vi "Resize Bounds.vi"(10 "Resize Amount":i16, 11 "Bounds In":T1) -> (3 "Bounds Out":T1)   [LabVIEW 2019, in "2D.lvlib"]
doc: "Resizes the bounding rectangle by the given amount. All edges of the rectangle will be changed by the Resize Amount. For example a resizing a bounding rectangle of [0,0,100,100] by 8 will result in a [-8,-8,108,108] bounding rectangle."
uses:
  <vilib>/Utility/miscctls.llb/LVRectTypeDef.ctl
  2D.lvlib
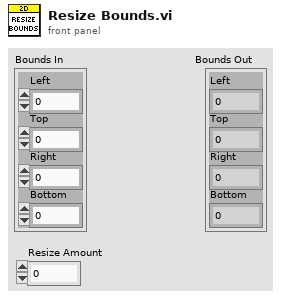
[diagram p1: front panel]
types:
  T1 = typedef "LVRectTypeDef.ctl" = cluster{"Left":i16, "Top":i16, "Right":i16, "Bottom":i16}
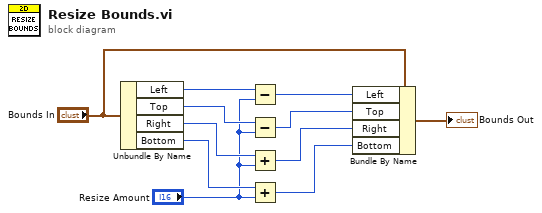
[diagram p0: block diagram]
diagram:
  n1 = Unbundle By Name("Bounds In") -> ("Left"=w9:i16, "Top"=w8:i16, "Right"=w11:i16, "Bottom"=w10:i16)
  n2 = Subtract(x=w9, y="Resize Amount") -> (x-y=w5:i16)
  n3 = Subtract(x=w8, y="Resize Amount") -> (x-y=w4:i16)
  n4 = Add(x=w11, y="Resize Amount") -> (x+y=w3:i16)
  n5 = Add(x=w10, y="Resize Amount") -> (x+y=w2:i16)
  n6 = Bundle By Name(cluster="Bounds In", "Left"=w5, "Top"=w4, "Right"=w3, "Bottom"=w2) -> (→"Bounds Out":T1)
